vi "MC AOTF Engine.vi"(0 "Notifier Name":string, 11 "Ports (Unused)":string[](array[string])) -> ()   [LabVIEW 2025]
uses:
  AOTF Controls/AOTF Notifier Element.ctl
  AOTF Controls/AOTF Actions.ctl
  AOTF Controls/AOTF Lines Lines Control.ctl
  <vilib>/ULx/Create Channel.llb/ULx Create Channel (DO-Digital Output).vi
  <vilib>/ULx/Write.llb/ULx Write (Digital Bool 1Line 1Point).vi
  <vilib>/ULx/Create Channel.llb/ULx Create Channel (AO-Voltage-Basic).vi
  <vilib>/ULx/Write.llb/ULx Write (Analog 1D DBL 1Chan 1Samp).vi
panel:
  in  "642 On":bool
  in  "560 On":bool
  in  "546 On":bool
  in  "488 On":bool
  in  "405 On":bool
  in  "Blank":bool
  in  "Quit":bool
  in  "546":dbl(slide) scale=0.0..100.0
  in  "642":dbl(slide) scale=0.0..100.0
  in  "560":dbl(slide) scale=0.0..100.0
  in  "488":dbl(slide) scale=0.0..100.0
  in  "405":dbl(slide) scale=0.0..100.0
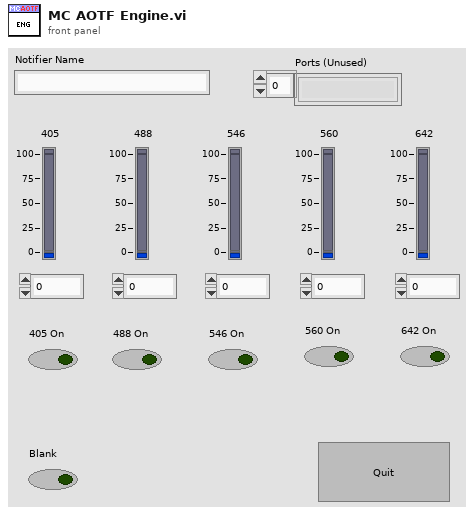
[diagram p1: front panel]
types:
  T1 = typedef "AOTF Lines Lines Control.ctl" = cluster{"Wavelength":u16[], "AO Line":string[]}
  T2 = typedef "AOTF Notifier Element.ctl" = cluster{"AOTF Action":T3, "Laser Line":string, "Power (%)":dbl, "Beam Blank On/Off":bool, "Line On/Off":bool, "Error":errorcluster, "Wavelengths (nm)":string[]}
  T3 = typedef "AOTF Actions.ctl" = enum16{"Error Check", "Blank", "Line On/Off", "Set Power", "Status", "Quit"}
  T4 = enum32{"Invalid", "Standard", "Closed", "Hidden", "Minimized", "Maximized"}
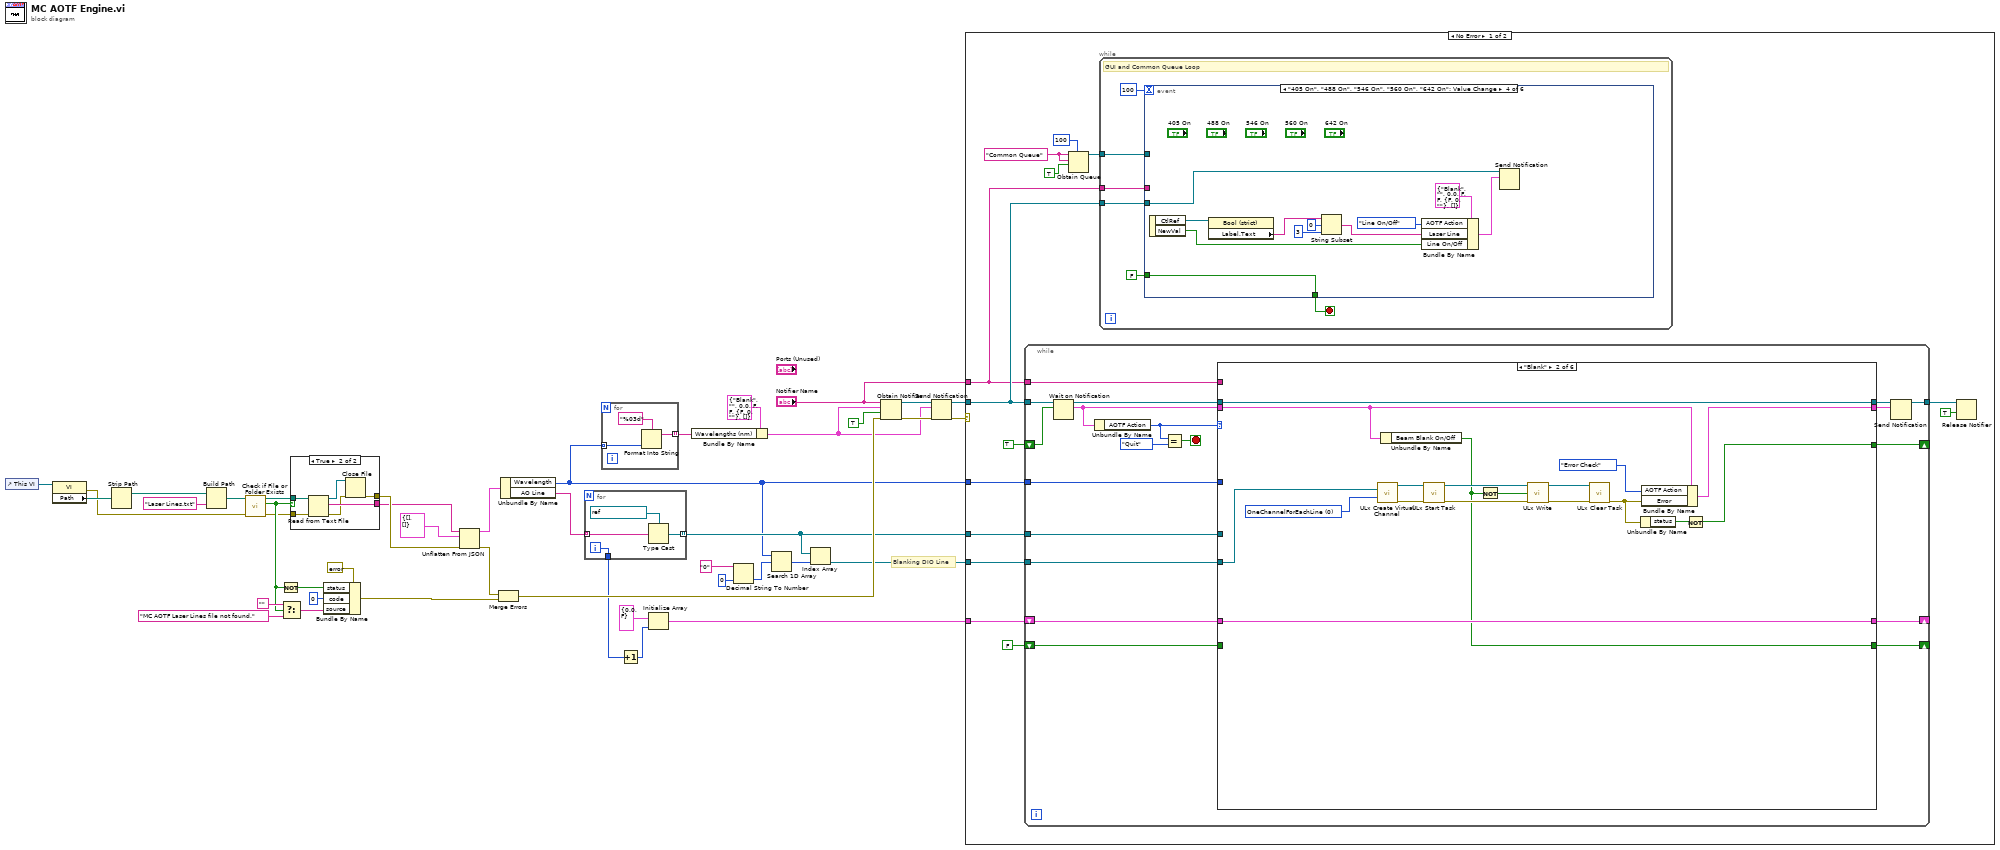
[diagram p0: block diagram]
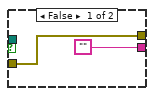
[diagram p2: hidden frame]
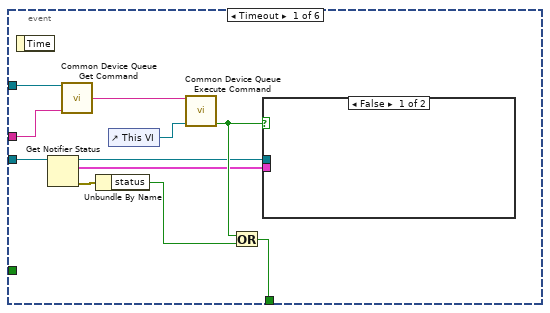
[diagram p3: hidden frame]
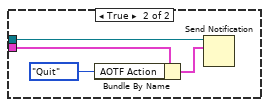
[diagram p4: hidden frame]
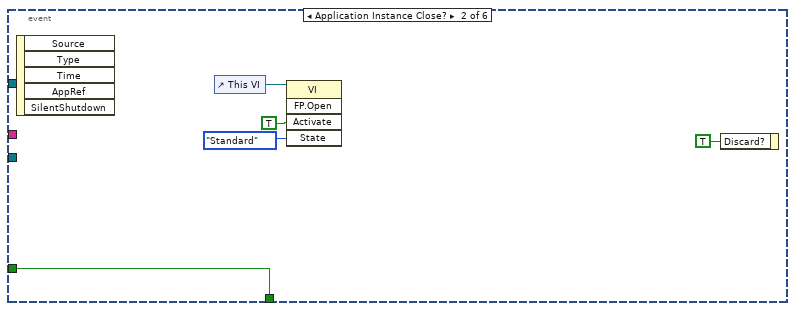
[diagram p5: hidden frame]
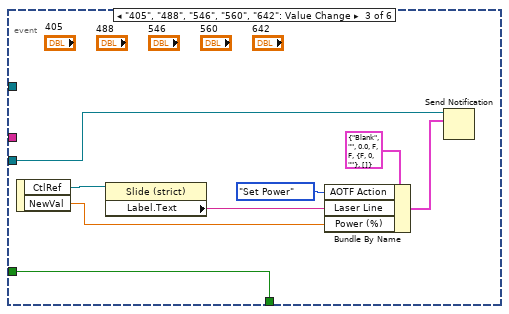
[diagram p6: hidden frame]
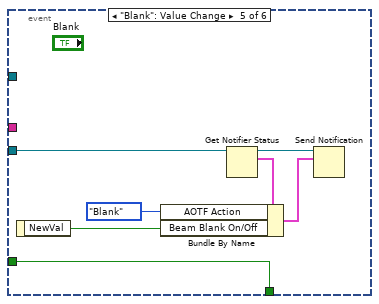
[diagram p7: hidden frame]
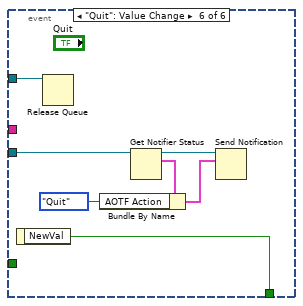
[diagram p8: hidden frame]
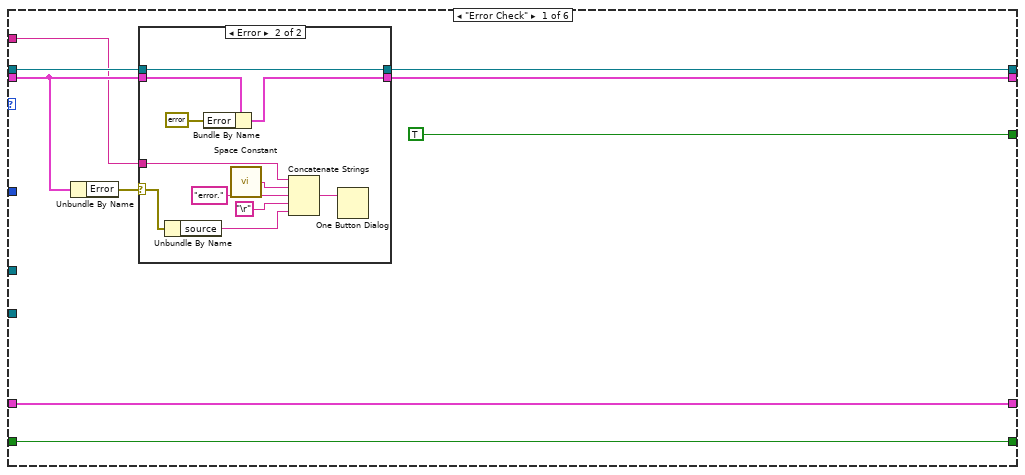
[diagram p9: hidden frame]
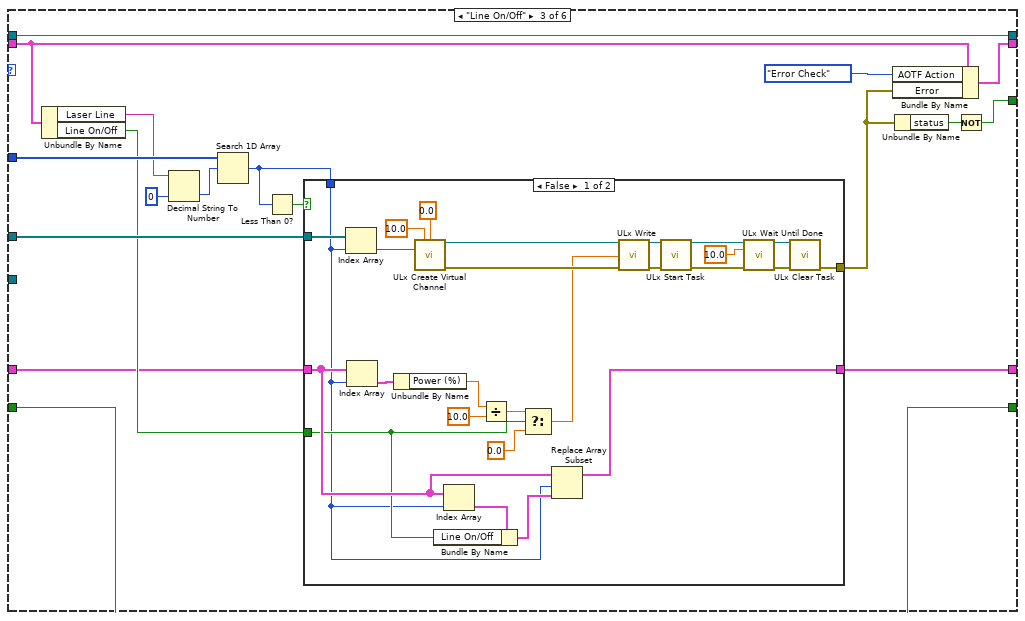
[diagram p11: hidden frame]
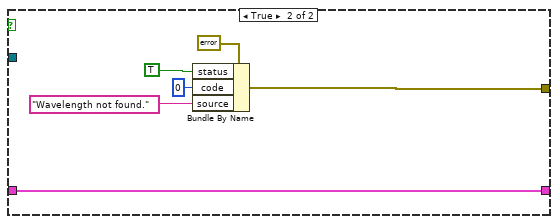
[diagram p12: hidden frame]
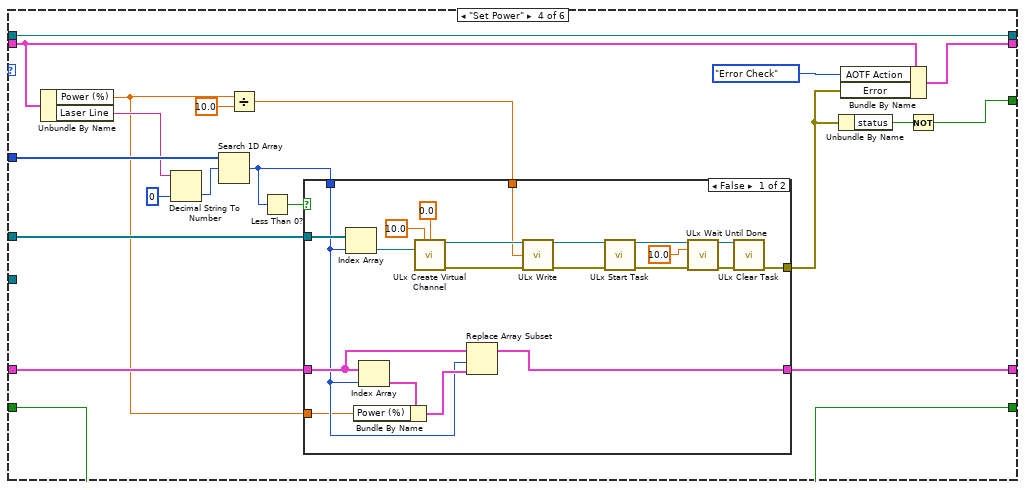
[diagram p13: hidden frame]
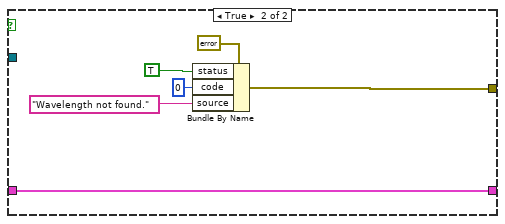
[diagram p14: hidden frame]
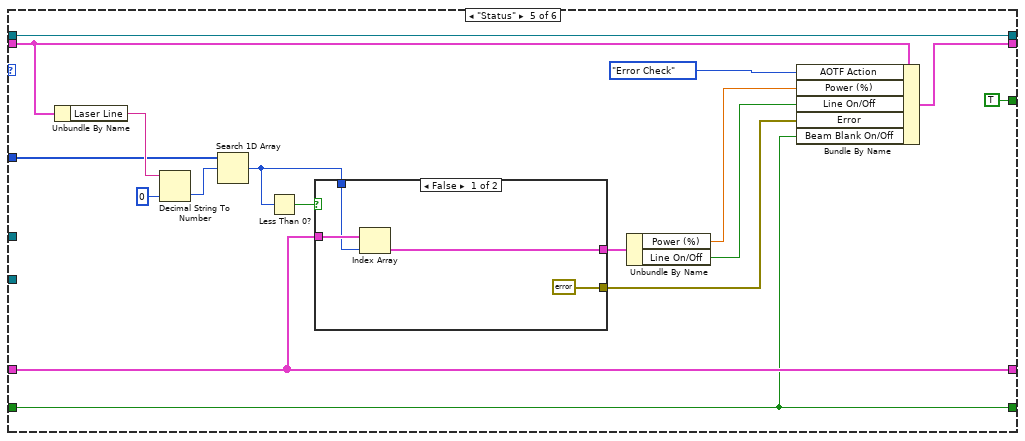
[diagram p15: hidden frame]
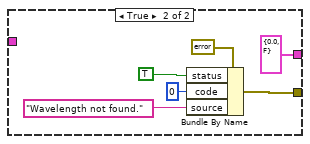
[diagram p16: hidden frame]
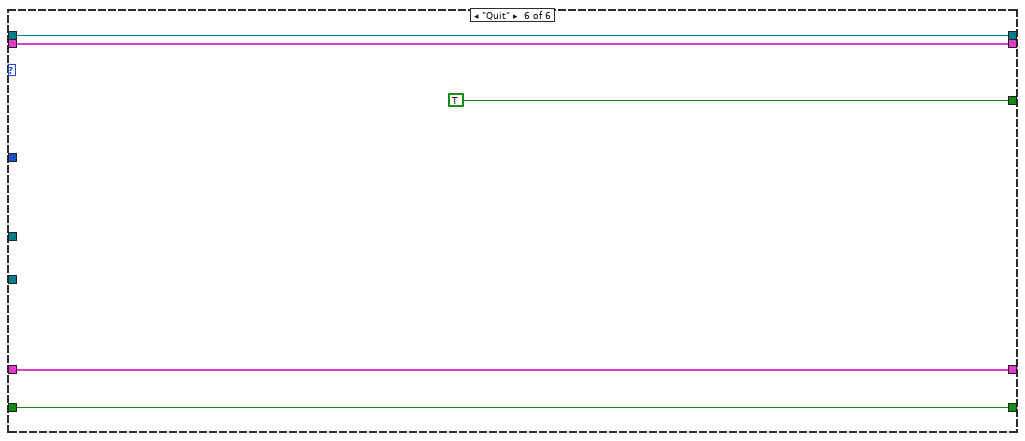
[diagram p17: hidden frame]
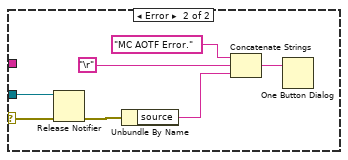
[diagram p18: hidden frame]
diagram:
  # "Blanking DIO Line"
  n1 = control-ref of="This VI"() -> (w42:refnum<vi>)
  n2 = property class="VI"(reference=w42) -> (error out=w28:errorcluster, "Path"=w41:path)  [unwired: 1 in, 1 out]
  n3 = Strip Path(path=w41) -> (stripped path=w40:path)  [unwired: 1 out]
  n4 = Build Path(base path=w40, name or relative path="Laser Lines.txt") -> (appended path=w38:path)
  n5 = call <vilib>:"Check if File or Folder Exists.vi"("error in (no error)"=w28, "path"=w38) -> ("error out"=w27:errorcluster, "file or folder exists?"=w30:bool, "dup path"=w29:path)  [unwired: 7 in]
  n6 = Not(x=w30) -> (.not. x?=w35:bool)
  n7 = Select(t="", s=w30, f="MC AOTF Laser Lines file not found." ("source")) -> (s? t:f=w31:string)
  n8 = case shown="True" w30 {
    tunnel: w29 -> [_ w51]
    tunnel: ["" w50] -> w22
    tunnel: w27 -> [w44 w48]
    tunnel: [w44 w46] -> w26
    frame False {
    }
    frame True {
      n9 = Read from Text File(file (use dialog)=w51, error in=w48) -> (refnum out=w49:refnum<file>, text=w50:string, error out=w47:errorcluster)  [unwired: 2 in, 1 out]
      n10 = Close File(refnum=w49, error in=w47) -> (error out=w46:errorcluster)  [unwired: 1 out]
    }
  }
  n11 = Bundle By Name(cluster=errorcluster {"status"=FALSE, "code"=0, "source"=""} ("Error"), "status"=w35, "code"=0, "source"=w31) -> (w24:errorcluster)
  n12 = Unflatten From JSON(JSON string=w22, type and defaults=T1 {"Wavelength"=[], "AO Line"=[]} ("Laser Lines"), error in (no error)=w26) -> (value=w20:T1, error out=w25:errorcluster)  [unwired: 4 in]
  n13 = Merge Errors(w25, w24) -> (w23:errorcluster)
  n14 = Unbundle By Name(w20) -> ("Wavelength"=w4:u16[], "AO Line"=w19:string[])
  n15 = for {
    tunnel: w19 -> [w54] mode=indexing
    tunnel: [w53] -> w15 mode=indexing
    tunnel: [w52] -> w10
    i -> [w52]
    n16 = Type Cast(type=refnum<k21> "Dev0/Ao12" ("Type Thingy"), x=w54) -> (*(type *) &x=w53:refnum<k21>)
  }
  n17 = for {
    tunnel: w4 -> [w58] mode=indexing
    tunnel: [w57] -> w2 mode=indexing
    n18 = Format Into String(format string="%03d", w58) -> (resulting string=w57:string)  [unwired: 2 in, 1 out]
  }
  n19 = Increment(x=w10) -> (x+1=w11:i32)
  n20 = Initialize Array(cluster{"Power (%)":dbl, "Line On/Off":bool} {"Power (%)"=0.0, "Line On/Off"=FALSE} ("Line Staus Cluster"), w11) -> (w9:cluster{"Power (%)":dbl, "Line On/Off":bool}[])
  n21 = Bundle By Name(cluster=T2 {"AOTF Action"=enum."Blank", "Laser Line"="", "Power (%)"=0.0, "Beam Blank On/Off"=FALSE, "Line On/Off"=FALSE, "Error"={"status"=FALSE, "code"=0, "source"=""}, "Wavelengths (nm)"=[]} ("AOTFQueueCtrl"), "Wavelengths (nm)"=w2) -> (w1:T2)
  n22 = Decimal String To Number(string="0", default (0L)=u16 0 ("default (0 I32)")) -> (number=w16:u16)  [unwired: 1 in, 1 out]
  n23 = Search 1D Array(1D array=w4, element=w16) -> (index of element=w14:i32)  [unwired: 1 in]
  n24 = Index Array(array=w15, index=w14) -> (element=w13:refnum<k21>)
  n25 = Obtain Notifier(name (unnamed)="Notifier Name", notification data type=w1, create if not found? (T)=TRUE, error in (no error)=w23) -> (notifier out=w8:refnum<notifier>, error out=w6:errorcluster)  [unwired: 1 out]
  n26 = Send Notification(notification=w1, notifier=w8, error in (no error)=w6) -> (notifier out=w7:refnum<notifier>, error out=w5:errorcluster)
  n27 = case shown="No Error" w5 {
    selector: w5 -> [_ w325]
    tunnel: w7 -> [w68 w326]
    tunnel: "Notifier Name" -> [w64 _]
    tunnel: w4 -> [w63 _]
    tunnel: w15 -> [w62 _]
    tunnel: w13 -> [w61 _]
    tunnel: w9 -> [w59 _]
    frame No Error {
      w72 = "Common Queue" ("Unique Notifier Name")
      n28 = while {
        tunnel: w68 -> [w150]
        shift-right: [w141] -> _
        shift-left: TRUE ("ignore previous (F)") -> [w149]
        tunnel: [w140] -> w66
        tunnel: w64 -> [w139]
        tunnel: w63 -> [w138]
        tunnel: w62 -> [w137]
        tunnel: w61 -> [w136]
        shift-right: [w132] -> _
        shift-left: FALSE -> [w133]
        shift-right: [w134] -> _
        shift-left: w59 -> [w135]
        stop <- w144 stop-if-true
        n29 = Wait on Notification(notifier=w150, ignore previous (F)=w149) -> (notifier out=w148:refnum<notifier>, notification=w147:T2)  [unwired: 2 in, 2 out]
        n30 = Unbundle By Name(w147) -> ("AOTF Action"=w146:T3)
        n31 = Equal?(x=w146, y=AOTF_Actions."Quit") -> (x = y?=w144:bool)
        n32 = case shown="\"Blank\"" w146 {
          tunnel: w148 -> [w159 w183 w206 w258 w304 w319]
          tunnel: w147 -> [w157 w182 w199 w249 w290 w318]
          tunnel: [w155 w183 w206 w258 w304 w319] -> w143
          tunnel: [w154 w181 w198 w248 w292 w318] -> w142
          tunnel: [TRUE w177 w197 w247 TRUE TRUE] -> w141
          tunnel: w139 -> [w156 _ _ _ _ _]
          tunnel: w138 -> [_ _ w208 w260 w293 _]
          tunnel: w137 -> [_ _ w207 w259 _ _]
          tunnel: w136 -> [_ w176 _ _ _ _]
          tunnel: w135 -> [w152 w175 w192 w244 w289 w316]
          tunnel: [w152 w175 w191 w243 w289 w316] -> w134
          tunnel: w133 -> [w151 _ w193 w242 w288 w315]
          tunnel: [w151 w174 w193 w242 w288 w315] -> w132
          frame "Error Check" {
            n33 = Unbundle By Name(w157) -> ("Error"=w158:errorcluster)
            n34 = case shown="Error" w158 {
              selector: w158 -> [_ w165]
              tunnel: w157 -> [w160 w169]
              tunnel: [w161 w167] -> w155
              tunnel: w159 -> [w161 w167]
              tunnel: w156 -> [_ w164]
              tunnel: [w160 w166] -> w154
              frame No Error {
              }
              frame Error {
                n35 = Unbundle By Name(w165) -> ("source"=w163:string)
                n36 = Bundle By Name(cluster=w169, "Error"=errorcluster {"status"=FALSE, "code"=0, "source"=""}) -> (w166:T2)
                n37 = call <vilib>:"Space Constant.vi"() -> ("String"=w172:string)
                n38 = Concatenate Strings(w164, w172, "error." ("string"), "\r", w163) -> (w170:string)
                n39 = One Button Dialog(message=w170) -> ()  [unwired: 1 in, 1 out]
              }
            }
          }
          frame "Blank" {
            w184 = 0 items=["OneChannelForEachLine", "OneChannelForAllLines"] ("line grouping")
            n40 = call-poly <vilib>:"ULx Create Virtual Channel.vi"("lines"=w176, "line grouping"=w184) -> ("task out"=w185:refnum<k24>, "error out"=w186:errorcluster)  [unwired: 12 in]
            n41 = Unbundle By Name(w182) -> ("Beam Blank On/Off"=w174:bool)
            n42 = call <vilib>:"ULx Start Task.vi"("task in"=w185, "error in"=w186) -> ("task out"=w187:refnum<k24>, "error out"=w188:errorcluster)  [unwired: 12 in]
            n43 = Not(x=w174) -> (.not. x?=w173:bool)
            n44 = call-poly <vilib>:"ULx Write.vi"("task in"=w187, "data"=w173, "error in"=w188) -> ("task out"=w189:refnum<k24>, "error out"=w190:errorcluster)  [unwired: 10 in, 1 out]
            n45 = call <vilib>:"ULx Clear Task.vi"("task in"=w189, "error in"=w190) -> ("error out"=w179:errorcluster)  [unwired: 13 in]
            n46 = Unbundle By Name(w179) -> ("status"=w178:bool)
            n47 = Bundle By Name(cluster=w182, "AOTF Action"=AOTF_Actions."Error Check", "Error"=w179) -> (w181:T2)
            n48 = Not(x=w178) -> (.not. x?=w177:bool)
          }
          frame "Line On/Off" {
            n49 = Unbundle By Name(w199) -> ("Laser Line"=w205:string, "Line On/Off"=w194:bool)
            n50 = Decimal String To Number(string=w205, default (0L)=u16 0 ("default (0 I32)")) -> (number=w203:u16)  [unwired: 1 in, 1 out]
            n51 = Search 1D Array(1D array=w208, element=w203) -> (index of element=w195:i32)  [unwired: 1 in]
            n52 = Less Than 0?(x=w195) -> (x < 0?=w196:bool)
            n53 = case shown="False" w196 {
              tunnel: w207 -> [w234 _]
              tunnel: [w222 w236] -> w200
              tunnel: w195 -> [w210 _]
              tunnel: w192 -> [w212 w235]
              tunnel: w194 -> [w211 _]
              tunnel: [w209 w235] -> w191
              frame False {
                n54 = Index Array(array=w234, index=w210) -> (element=w223:refnum<k21>)
                n55 = Index Array(array=w212, index=w210) -> (element=w220:cluster{"Power (%)":dbl, "Line On/Off":bool})
                n56 = Unbundle By Name(w220) -> ("Power (%)"=w217:dbl)
                n57 = call-poly <vilib>:"ULx Create Virtual Channel.vi"("maximum value"=10.0, "minimum value"=0.0, "physical channels"=w223) -> ("task out"=w233:refnum<k24>, "error out"=w226:errorcluster)  [unwired: 11 in]
                n58 = Index Array(array=w212, index=w210) -> (element=w214:cluster{"Power (%)":dbl, "Line On/Off":bool})
                n59 = Bundle By Name(cluster=w214, "Line On/Off"=w211) -> (w213:cluster{"Power (%)":dbl, "Line On/Off":bool})
                n60 = Divide(x=w217, y=10.0) -> (x/y=w216:dbl)
                n61 = Select(t=w216, s=w211, f=0.0 ("minimum value")) -> (s? t:f=w215:dbl)
                n62 = Replace Array Subset(array=w212, new element=w213, index=w210) -> (w209:cluster{"Power (%)":dbl, "Line On/Off":bool}[])
                n63 = call-poly <vilib>:"ULx Write.vi"("task in"=w233, "data"=w215, "error in"=w226) -> ("task out"=w221:refnum<k24>, "error out"=w227:errorcluster)  [unwired: 10 in, 1 out]
                n64 = call <vilib>:"ULx Start Task.vi"("task in"=w221, "error in"=w227) -> ("task out"=w232:refnum<k24>, "error out"=w229:errorcluster)  [unwired: 12 in]
                n65 = call <vilib>:"ULx Wait Until Done.vi"("task in"=w232, "timeout"=10.0, "error in"=w229) -> ("task out"=w231:refnum<k24>, "error out"=w228:errorcluster)  [unwired: 11 in]
                n66 = call <vilib>:"ULx Clear Task.vi"("task in"=w231, "error in"=w228) -> ("error out"=w222:errorcluster)  [unwired: 13 in]
              }
              frame True {
                n67 = Bundle By Name(cluster=errorcluster {"status"=FALSE, "code"=0, "source"=""} ("error out"), "status"=TRUE, "code"=0, "source"="Wavelength not found.") -> (w236:errorcluster)
              }
            }
            n68 = Bundle By Name(cluster=w199, "AOTF Action"=AOTF_Actions."Error Check", "Error"=w200) -> (w198:T2)
            n69 = Unbundle By Name(w200) -> ("status"=w201:bool)
            n70 = Not(x=w201) -> (.not. x?=w197:bool)
          }
          frame "Set Power" {
            n71 = Unbundle By Name(w249) -> ("Power (%)"=w241:dbl, "Laser Line"=w257:string)
            n72 = Decimal String To Number(string=w257, default (0L)=u16 0 ("default (0 I32)")) -> (number=w255:u16)  [unwired: 1 in, 1 out]
            n73 = Search 1D Array(1D array=w260, element=w255) -> (index of element=w245:i32)  [unwired: 1 in]
            n74 = Divide(x=w241, y=10.0) -> (x/y=w253:dbl)
            n75 = Less Than 0?(x=w245) -> (x < 0?=w246:bool)
            n76 = case shown="False" w246 {
              tunnel: w259 -> [w281 _]
              tunnel: w253 -> [w269 _]
              tunnel: [w268 w283] -> w250
              tunnel: w245 -> [w263 _]
              tunnel: w244 -> [w264 w282]
              tunnel: [w262 w282] -> w243
              tunnel: w241 -> [w261 _]
              frame False {
                n77 = Index Array(array=w281, index=w263) -> (element=w270:refnum<k21>)
                n78 = Index Array(array=w264, index=w263) -> (element=w266:cluster{"Power (%)":dbl, "Line On/Off":bool})
                n79 = Bundle By Name(cluster=w266, "Power (%)"=w261) -> (w265:cluster{"Power (%)":dbl, "Line On/Off":bool})
                n80 = call-poly <vilib>:"ULx Create Virtual Channel.vi"("maximum value"=10.0, "minimum value"=0.0, "physical channels"=w270) -> ("task out"=w280:refnum<k24>, "error out"=w273:errorcluster)  [unwired: 11 in]
                n81 = Replace Array Subset(array=w264, new element=w265, index=w263) -> (w262:cluster{"Power (%)":dbl, "Line On/Off":bool}[])
                n82 = call-poly <vilib>:"ULx Write.vi"("task in"=w280, "data"=w269, "error in"=w273) -> ("task out"=w267:refnum<k24>, "error out"=w274:errorcluster)  [unwired: 10 in, 1 out]
                n83 = call <vilib>:"ULx Start Task.vi"("task in"=w267, "error in"=w274) -> ("task out"=w279:refnum<k24>, "error out"=w276:errorcluster)  [unwired: 12 in]
                n84 = call <vilib>:"ULx Wait Until Done.vi"("task in"=w279, "timeout"=10.0, "error in"=w276) -> ("task out"=w278:refnum<k24>, "error out"=w275:errorcluster)  [unwired: 11 in]
                n85 = call <vilib>:"ULx Clear Task.vi"("task in"=w278, "error in"=w275) -> ("error out"=w268:errorcluster)  [unwired: 13 in]
              }
              frame True {
                n86 = Bundle By Name(cluster=errorcluster {"status"=FALSE, "code"=0, "source"=""} ("error out"), "status"=TRUE, "code"=0, "source"="Wavelength not found.") -> (w283:errorcluster)
              }
            }
            n87 = Unbundle By Name(w250) -> ("status"=w251:bool)
            n88 = Bundle By Name(cluster=w249, "AOTF Action"=AOTF_Actions."Error Check", "Error"=w250) -> (w248:T2)
            n89 = Not(x=w251) -> (.not. x?=w247:bool)
          }
          frame "Status" {
            n90 = Unbundle By Name(w290) -> ("Laser Line"=w296:string)
            n91 = Decimal String To Number(string=w296, default (0L)=u16 0 ("default (0 I32)")) -> (number=w295:u16)  [unwired: 1 in, 1 out]
            n92 = Search 1D Array(1D array=w293, element=w295) -> (index of element=w298:i32)  [unwired: 1 in]
            n93 = Less Than 0?(x=w298) -> (x < 0?=w297:bool)
            n94 = case shown="False" w297 {
              tunnel: w289 -> [w308 _]
              tunnel: [errorcluster {"status"=FALSE, "code"=0, "source"=""} ("error out") w310] -> w300
              tunnel: w298 -> [w307 _]
              tunnel: [w306 cluster{"Power (%)":dbl, "Line On/Off":bool} {"Power (%)"=0.0, "Line On/Off"=FALSE} ("Line Staus Cluster")] -> w301
              frame False {
                n95 = Index Array(array=w308, index=w307) -> (element=w306:cluster{"Power (%)":dbl, "Line On/Off":bool})
              }
              frame True {
                n96 = Bundle By Name(cluster=errorcluster {"status"=FALSE, "code"=0, "source"=""} ("error out"), "status"=TRUE, "code"=0, "source"="Wavelength not found.") -> (w310:errorcluster)
              }
            }
            n97 = Unbundle By Name(w301) -> ("Power (%)"=w302:dbl, "Line On/Off"=w303:bool)
            n98 = Bundle By Name(cluster=w290, "AOTF Action"=AOTF_Actions."Error Check", "Power (%)"=w302, "Line On/Off"=w303, "Error"=w300, "Beam Blank On/Off"=w288) -> (w292:T2)
          }
          frame "Quit" {
          }
        }
        n99 = Send Notification(notification=w142, notifier=w143) -> (notifier out=w140:refnum<notifier>)  [unwired: 1 in, 1 out]
      }
      n100 = Obtain Queue(max queue size (-1, unlimited)=100, name (unnamed)=w72, element data type=w72, create if not found? (T)=TRUE) -> (queue out=w69:refnum<queue>)  [unwired: 1 in, 2 out]
      n101 = while {
        tunnel: w69 -> [w77]
        tunnel: w64 -> [w75]
        tunnel: w68 -> [w76]
        stop <- w74 stop-if-true
        # "GUI and Common Queue Loop"
        n102 = event shown="[3] \"405 On\", \"488 On\", \"546 On\", \"560 On\", \"642 On\": Value Change" {
          selector: _ -> [_ _ _ _ _ _]
          dyn-events: _ -> [_ _ _ _ _ _]
          timeout: 100 -> [_ _ _ _ _ _]
          tunnel: w77 -> [w84 _ _ _ _ w131]
          tunnel: w76 -> [w80 _ w105 w116 w123 w130]
          tunnel: w75 -> [w83 _ _ _ _ _]
          tunnel: [w82 w98 w106 w117 w124 w128] -> w74
          tunnel: FALSE -> [_ w98 w106 w117 w124 _]
          event Timeout {
            n103 = event-data() -> ()  [unwired: 1 in, 1 out]
            n104 = Get Notifier Status(notifier=w80) -> (notifier out=w79:refnum<notifier>, current notification=w81:T2, error out=w89:errorcluster)  [unwired: 1 in, 2 out]
            n105 = call "Common Device Queue Get Command.vi"("Common Queue"=w84, "Notifier Name"=w83) -> ("Command"=w88:string)  [unwired: 12 in, 1 out]
            n106 = Unbundle By Name(w89) -> ("status"=w86:bool)
            n107 = control-ref of="This VI"() -> (w87:refnum<vi>)
            n108 = call "Common Device Queue Execute Command.vi"("Common Command"=w88, "VI Refnum"=w87) -> ("Quit?"=w85:bool)  [unwired: 12 in, 1 out]
            n109 = Or(x=w85, y=w86) -> (x .or. y?=w82:bool)
            n110 = case shown="False" w85 {
              tunnel: w79 -> [_ w93]
              tunnel: w81 -> [_ w92]
              frame False {
              }
              frame True {
                n111 = Bundle By Name(cluster=w92, "AOTF Action"=AOTF_Actions."Quit") -> (w91:T2)
                n112 = Send Notification(notification=w91, notifier=w93) -> ()  [unwired: 1 in, 2 out]
              }
            }
          }
          event Application Instance Close? {
            n113 = event-data() -> ()  [unwired: 1 in, 5 out]
            n114 = control-ref of="This VI"() -> (w95:refnum<vi>)
            n115 = invoke class="VI" method="FP.Open"(reference=w95, "Activate"=TRUE ("Activate?"), "State"=T4."Standard") -> ()  [unwired: 2 in, 5 out]
            n116 = event-data("Discard?"=TRUE) -> ()  [unwired: 1 in, 1 out]
          }
          event "405", "488", "546", "560", "642": Value Change {
            n117 = event-data() -> ("CtlRef"=w104:refnum<vi>, "NewVal"=w100:dbl)  [unwired: 1 in]
            n118 = property class="Slide (strict)"(reference=w104) -> ("Label.Text"=w101:string)  [unwired: 1 in, 2 out]
            n119 = Bundle By Name(cluster=T2 {"AOTF Action"=enum."Blank", "Laser Line"="", "Power (%)"=0.0, "Beam Blank On/Off"=FALSE, "Line On/Off"=FALSE, "Error"={"status"=FALSE, "code"=0, "source"=""}, "Wavelengths (nm)"=[]} ("AOTFQueueCtrl"), "AOTF Action"=AOTF_Actions."Set Power", "Laser Line"=w101, "Power (%)"=w100) -> (w99:T2)
            n120 = Send Notification(notification=w99, notifier=w105) -> ()  [unwired: 1 in, 2 out]
          }
          event "405 On", "488 On", "546 On", "560 On", "642 On": Value Change {
            n121 = event-data() -> ("CtlRef"=w115:refnum<vi>, "NewVal"=w111:bool)  [unwired: 1 in]
            n122 = property class="Bool (strict)"(reference=w115) -> ("Label.Text"=w110:string)  [unwired: 1 in, 2 out]
            n123 = String Subset(string=w110, offset (0)=0, length (rest)=3 ("length (rest)")) -> (substring=w107:string)
            n124 = Bundle By Name(cluster=T2 {"AOTF Action"=enum."Blank", "Laser Line"="", "Power (%)"=0.0, "Beam Blank On/Off"=FALSE, "Line On/Off"=FALSE, "Error"={"status"=FALSE, "code"=0, "source"=""}, "Wavelengths (nm)"=[]} ("AOTFQueueCtrl"), "AOTF Action"=AOTF_Actions."Line On/Off", "Laser Line"=w107, "Line On/Off"=w111) -> (w112:T2)
            n125 = Send Notification(notification=w112, notifier=w116) -> ()  [unwired: 1 in, 2 out]
          }
          event "Blank": Value Change {
            n126 = event-data() -> ("NewVal"=w119:bool)  [unwired: 1 in]
            n127 = Get Notifier Status(notifier=w123) -> (notifier out=w122:refnum<notifier>, current notification=w121:T2)  [unwired: 1 in, 3 out]
            n128 = Bundle By Name(cluster=w121, "AOTF Action"=AOTF_Actions."Blank", "Beam Blank On/Off"=w119) -> (w118:T2)
            n129 = Send Notification(notification=w118, notifier=w122) -> ()  [unwired: 1 in, 2 out]
          }
          event "Quit": Value Change {
            n130 = event-data() -> ("NewVal"=w128:bool)  [unwired: 1 in]
            n131 = Release Queue(queue=w131) -> ()  [unwired: 2 in, 3 out]
            n132 = Get Notifier Status(notifier=w130) -> (notifier out=w129:refnum<notifier>, current notification=w127:T2)  [unwired: 1 in, 3 out]
            n133 = Bundle By Name(cluster=w127, "AOTF Action"=AOTF_Actions."Quit") -> (w125:T2)
            n134 = Send Notification(notification=w125, notifier=w129) -> ()  [unwired: 1 in, 2 out]
          }
        }
      }
      n135 = Release Notifier(notifier=w66, force destroy? (F)=TRUE) -> ()  [unwired: 1 in, 3 out]
    }
    frame Error {
      n136 = Release Notifier(notifier=w326, error in (no error)=w325) -> (error out=w322:errorcluster)  [unwired: 1 in, 2 out]
      n137 = Unbundle By Name(w322) -> ("source"=w321:string)
      n138 = Concatenate Strings("MC AOTF Error.", "\r", w321) -> (w320:string)
      n139 = One Button Dialog(message=w320) -> ()  [unwired: 1 in, 1 out]
    }
  }
